vi "Add Child.vi"(8 "error in (no error)":errorcluster, 9 "name":string, 10 "child":refnum<class "Type Definition.lvclass">, 11 "Type Definition in":refnum<class "Type Definition.lvclass">) -> (0 "error out":errorcluster, 3 "Type Definition out":refnum<class "Type Definition.lvclass">)   [LabVIEW 2020, in "PV Access.lvlib" / "PV Data.lvlib" / "Type Definition.lvclass"]
uses:
  Type Definition.lvclass
  Type Definition.lvclass/Type Definition.ctl
  PV Access.lvlib
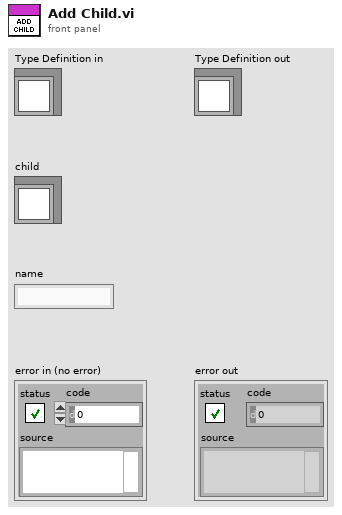
[diagram p1: front panel]
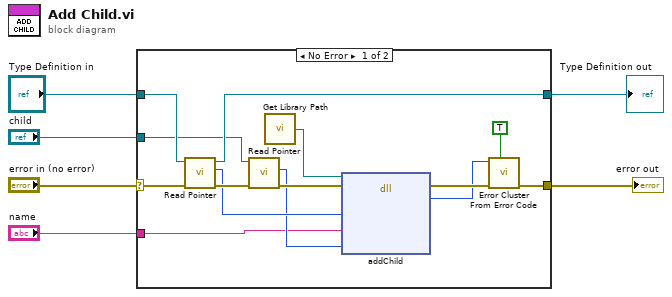
[diagram p0: block diagram]
diagram:
  n1 = case shown="No Error" "error in (no error)" {
    selector: "error in (no error)" -> [w18 w22]
    tunnel: [w9 w22] -> w5
    tunnel: [w13 w21] -> w3
    tunnel: "Type Definition in" -> [w14 w21]
    tunnel: "name" -> [w8 _]
    tunnel: "child" -> [w7 _]
    frame No Error {
      n2 = call-dynamic "Read Pointer.vi"("error in (no error)"=w18, "Pointer Base in"=w14) -> ("error out"=w19:errorcluster, "Pointer"=w16:i64, "Pointer Base out"=w13:refnum<class "Type Definition.lvclass">)  [unwired: 7 in]
      n3 = call-dynamic "Read Pointer.vi"("error in (no error)"=w19, "Pointer Base in"=w7) -> ("error out"=w17:errorcluster, "Pointer"=w15:i64)  [unwired: 7 in, 1 out]
      n4 = call "Get Library Path.vi"() -> ("Path"=w20:path)  [unwired: 1 in]
      n5 = dll-call lib="?" fn="addChild"(path in=w20, error in=w17, "type def"=w16, "name"=w8, "child"=w15) -> (error out=w11:errorcluster, "err_code"=w10:i32)  [unwired: 4 in, 1 out]
      n6 = call <vilib>:"Error Cluster From Error Code.vi"("show call chain? (False)"=TRUE, "error in (no error)"=w11, "error code (0)"=w10) -> ("error out"=w9:errorcluster)  [unwired: 6 in]
    }
    frame Error {
    }
  }
  "error out" <- w5
  "Type Definition out" <- w3
